vi "Calc Dist to ConstV.vi"(9 "V2 (fps)":dbl=10.0, 10 "Limits":T2={"Acceleration (fps^2)"=10.0, "Jerk (fps^3)"=100.0}, 11 "V1  (fps)":dbl) -> (1 "distances":T1, 2 "Time to const V":dbl, 3 "distance (ft)":dbl)   [LabVIEW 2019]
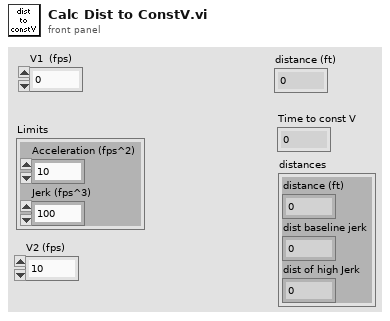
[diagram p1: front panel]
types:
  T1 = cluster{"distance (ft)":dbl, "dist baseline jerk":dbl, "dist of high Jerk":dbl}
  T2 = cluster{"Acceleration (fps^2)":dbl, "Jerk (fps^3)":dbl}
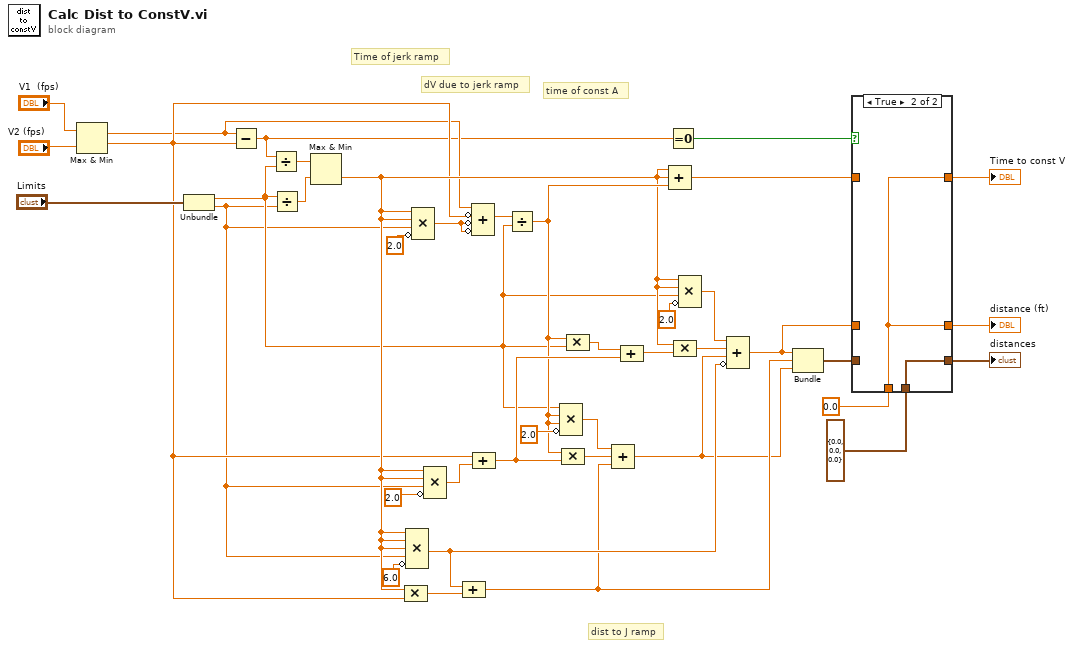
[diagram p0: block diagram]
diagram:
  # "dist to J ramp"
  # "time of const A"
  # "dV due to jerk ramp"
  # "Time of jerk ramp"
  n1 = Max & Min(x="V1  (fps)", y="V2 (fps)") -> (max(x,y)=w13:dbl, min(x,y)=w14:dbl)
  n2 = Unbundle("Limits") -> ("Acceleration (fps^2)"=w12:dbl, "Jerk (fps^3)"=w11:dbl)
  n3 = Subtract(x=w13, y=w14) -> (x-y=w10:dbl)
  n4 = Divide(x=w10, y=w12) -> (x/y=w21:dbl)
  n5 = Divide(x=w12, y=w11) -> (x/y=w20:dbl)
  n6 = Max & Min(x=w21, y=w20) -> (min(x,y)=w19:dbl)  [unwired: 1 out]
  n7 = Compound Arithmetic op=MULTIPLY(w19, w14) -> (w34:dbl)
  n8 = Compound Arithmetic op=MULTIPLY(w19, w19, w19, w11, invert 6.0) -> (w25:dbl)
  n9 = Compound Arithmetic op=MULTIPLY(w19, w19, w11, invert 2.0) -> (w35:dbl)
  n10 = Compound Arithmetic op=MULTIPLY(w19, w19, w11, invert 2.0) -> (w24:dbl)
  n11 = Compound Arithmetic op=ADD(w25, w34) -> (w18:dbl)
  n12 = Compound Arithmetic op=ADD(w13, invert w14, invert w35, invert w35) -> (w38:dbl)
  n13 = Compound Arithmetic op=ADD(w14, w24) -> (w29:dbl)
  n14 = Divide(x=w38, y=w12) -> (x/y=w28:dbl)
  n15 = Compound Arithmetic op=MULTIPLY(w12, w28, w28, invert 2.0) -> (w32:dbl)
  n16 = Compound Arithmetic op=MULTIPLY(w28, w29) -> (w33:dbl)
  n17 = Compound Arithmetic op=MULTIPLY(w28, w12) -> (w27:dbl)
  n18 = Compound Arithmetic op=ADD(w32, w33, w18) -> (w17:dbl)
  n19 = Compound Arithmetic op=ADD(w27, w29) -> (w26:dbl)
  n20 = Equal To 0?(x=w10) -> (x = 0?=w9:bool)
  n21 = Compound Arithmetic op=ADD(w19, w19, w28) -> (w8:dbl)
  n22 = Compound Arithmetic op=MULTIPLY(w19, w26) -> (w31:dbl)
  n23 = Compound Arithmetic op=MULTIPLY(w19, w19, w12, invert 2.0) -> (w22:dbl)
  n24 = Compound Arithmetic op=ADD(w22, w31, w17, invert w25) -> (w7:dbl)
  n25 = Bundle(w7, w18, w17) -> (w6:cluster{dbl, dbl, dbl})  [unwired: 1 in]
  n26 = case shown="True" w9 {
    tunnel: w8 -> [w41 _]
    tunnel: w7 -> [w42 _]
    tunnel: w6 -> [w43 _]
    tunnel: [w43 w45] -> w5
    tunnel: [w42 w44] -> w4
    tunnel: [w41 w44] -> w3
    tunnel: cluster{dbl, dbl, dbl} {0.0, 0.0, 0.0} ("output cluster") -> [_ w45]
    tunnel: 0.0 -> [_ w44]
    frame False {
    }
    frame True {
    }
  }
  "Time to const V" <- w3
  "distances" <- w5
  "distance (ft)" <- w4
